vi "FK.vi"(8 "error in (no error)":errorcluster, 10 "joints":dbl[](array[numeric]), 11 "Delta Robot Kinematics in":refnum<class "Delta Robot Kinematics.lvclass">) -> (0 "error out":errorcluster, 1 "exist":bool, 2 "p":dbl[](array[numeric]), 3 "Delta Robot Kinematics out":refnum<class "Delta Robot Kinematics.lvclass">)   [LabVIEW 2014, in "Delta Robot Kinematics.lvclass"]
uses:
  Delta Robot Kinematics.lvclass
  Delta Robot Kinematics.lvclass/Delta Robot Kinematics.ctl
  <vilib>/Analysis/baseanly.llb/A x Vector.vi
  <vilib>/Analysis/_algsub.llb/Real Vector Norm.vi
  <vilib>/Analysis/baseanly.llb/Outer Product.vi
  <vilib>/Analysis/baseanly.llb/Real Outer Product.vi
  <vilib>/robotics/Kinematics/Create Lie Group Matrix.vi
  <vilib>/Analysis/7linalg.llb/Create Special Matrix.vi
  <vilib>/Analysis/7linalg.llb/Create Special Real Matrix.vi
  <vilib>/Analysis/Matrix/Numeric/Multiply/Multiply.vi
  <vilib>/Analysis/Matrix/Numeric/Multiply/Multiply - RM,R.vi
  <vilib>/Analysis/Matrix/Numeric/Multiply/Multiply - R,RM.vi
  <vilib>/Analysis/Matrix/Numeric/Add/Add.vi
  <vilib>/Analysis/Matrix/Numeric/Add/Add - RM,RM.vi
  <vilib>/robotics/Kinematics/NI_Kinematics.lvlib
  <vilib>/Analysis/NI_AALBase.lvlib
  <vilib>/Analysis/NI_AALPro.lvlib
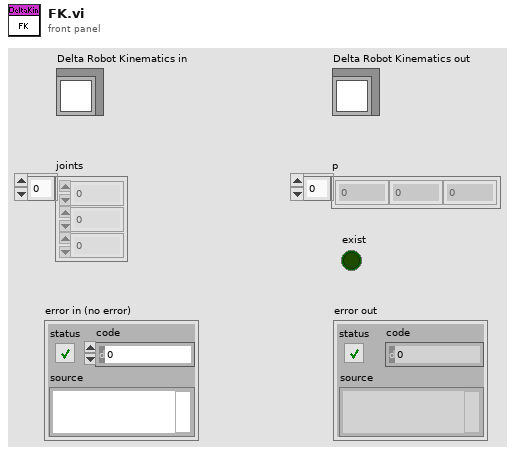
[diagram p1: front panel]
types:
  T1 = typedef "NI_Matrix.lvlib/RealMatrix.ctl" = dbl[][]
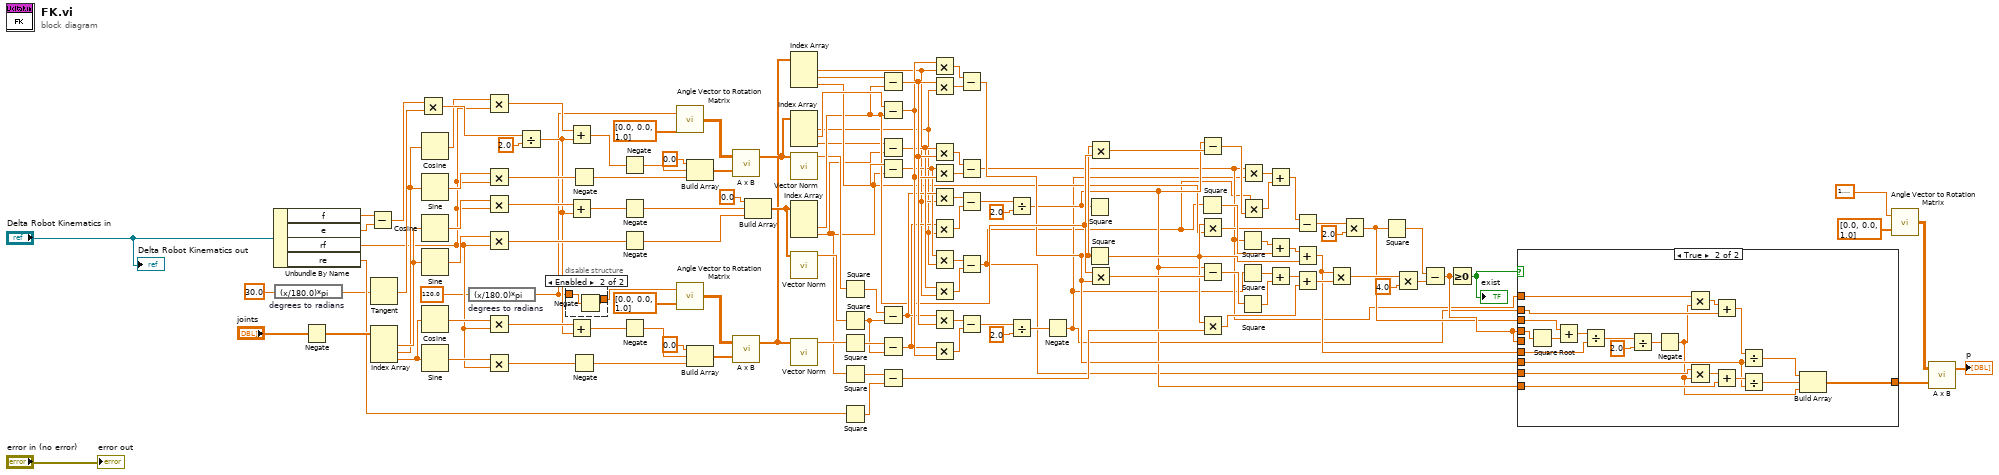
[diagram p0: block diagram]
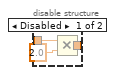
[diagram p2: hidden frame]
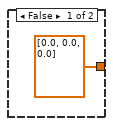
[diagram p3: hidden frame]
diagram:
  n1 = Unbundle By Name("Delta Robot Kinematics in") -> ("f"=w11:dbl, "e"=w10:dbl, "rf"=w9:dbl, "re"=w8:dbl)
  n2 = expression code="(x/180.0)*pi" "degrees to radians"(30.0) -> (w6:dbl)
  n3 = Negate(x="joints") -> (-x=w30:dbl[])
  n4 = Subtract(x=w11, y=w10) -> (x-y=w128:dbl)
  n5 = Tangent(1:w6) -> (0:w127:dbl)
  n6 = Index Array(array=w30) -> (element #1=w121:dbl, element #2=w51:dbl, element #3=w50:dbl)  [unwired: 3 in]
  n7 = Multiply(x=w128, y=w127) -> (x*y=w126:dbl)
  n8 = Cosine(x=w51) -> (cos(x)=w37:dbl)
  n9 = Sine(x=w51) -> (sin(x)=w35:dbl)
  n10 = Cosine(x=w121) -> (cos(x)=w124:dbl)
  n11 = Sine(x=w121) -> (sin(x)=w120:dbl)
  n12 = Cosine(x=w50) -> (cos(x)=w36:dbl)
  n13 = Sine(x=w50) -> (sin(x)=w33:dbl)
  n14 = expression code="(x/180.0)*pi" "degrees to radians"(120.0) -> (w4:dbl)
  n15 = Multiply(x=w37, y=w9) -> (x*y=w49:dbl)
  n16 = Multiply(x=w35, y=w9) -> (x*y=w47:dbl)
  n17 = Multiply(x=w124, y=w9) -> (x*y=w123:dbl)
  n18 = Multiply(x=w120, y=w9) -> (x*y=w119:dbl)
  n19 = Multiply(x=w36, y=w9) -> (x*y=w38:dbl)
  n20 = Multiply(x=w33, y=w9) -> (x*y=w40:dbl)
  n21 = Divide(x=w126, y=2.0) -> (x/y=w34:dbl)
  n22 = disable-structure shown="Enabled" {
    disable-tunnel: [w131 w133] -> w27
    disable-tunnel: w4 -> [w130 w134]
    frame Disabled {
      n23 = Multiply(x=w130, y=2.0) -> (x*y=w131:dbl)
    }
    frame Enabled {
      n24 = Negate(x=w134) -> (-x=w133:dbl)
    }
  }
  n25 = Add(x=w49, y=w34) -> (x+y=w48:dbl)
  n26 = Add(x=w123, y=w34) -> (x+y=w122:dbl)
  n27 = Add(x=w38, y=w34) -> (x+y=w39:dbl)
  n28 = Negate(x=w47) -> (-x=w45:dbl)
  n29 = Negate(x=w40) -> (-x=w42:dbl)
  n30 = Negate(x=w48) -> (-x=w46:dbl)
  n31 = Negate(x=w122) -> (-x=w118:dbl)
  n32 = Negate(x=w119) -> (-x=w117:dbl)
  n33 = Negate(x=w39) -> (-x=w41:dbl)
  n34 = call <vilib>:"Angle Vector to Rotation Matrix.vi"("vector"=dbl[] [0.0, 0.0, 1.0], "angle"=w4) -> ("rotation matrix"=w114:T1)
  n35 = call <vilib>:"Angle Vector to Rotation Matrix.vi"("vector"=dbl[] [0.0, 0.0, 1.0], "angle"=w27) -> ("rotation matrix"=w28:T1)
  n36 = Build Array(0.0 ("element"), w46, w45) -> (w32:dbl[])
  n37 = Build Array(0.0 ("element"), w41, w42) -> (w31:dbl[])
  n38 = call-poly <vilib>:"A x B.vi"("Vector"=w32, "A"=w114) -> ("A x Vector"=w108:dbl[])  [unwired: 1 out]
  n39 = call-poly <vilib>:"A x B.vi"("Vector"=w31, "A"=w28) -> ("A x Vector"=w107:dbl[])  [unwired: 1 out]
  n40 = Build Array(0.0 ("element"), w118, w117) -> (w109:dbl[])
  n41 = Index Array(array=w107) -> (element #1=w90:dbl, element #2=w111:dbl, element #3=w105:dbl)  [unwired: 3 in]
  n42 = Index Array(array=w108) -> (element #1=w19:dbl, element #2=w113:dbl, element #3=w20:dbl)  [unwired: 3 in]
  n43 = call-poly <vilib>:"Vector Norm.vi"("Input Vector"=w108) -> ("norm"=w24:dbl)  [unwired: 9 in, 1 out]
  n44 = Index Array(array=w109) -> (element #2=w75:dbl, element #3=w18:dbl)  [unwired: 3 in, 1 out]
  n45 = call-poly <vilib>:"Vector Norm.vi"("Input Vector"=w109) -> ("norm"=w22:dbl)  [unwired: 9 in, 1 out]
  n46 = call-poly <vilib>:"Vector Norm.vi"("Input Vector"=w107) -> ("norm"=w26:dbl)  [unwired: 9 in, 1 out]
  n47 = Square(x=w24) -> (x^2=w23:dbl)
  n48 = Square(x=w22) -> (x^2=w21:dbl)
  n49 = Square(x=w26) -> (x^2=w25:dbl)
  n50 = Square(x=w18) -> (x^2=w70:dbl)
  n51 = Square(x=w8) -> (x^2=w69:dbl)
  n52 = Subtract(x=w111, y=w75) -> (x-y=w103:dbl)
  n53 = Subtract(x=w113, y=w75) -> (x-y=w102:dbl)
  n54 = Subtract(x=w20, y=w18) -> (x-y=w96:dbl)
  n55 = Subtract(x=w105, y=w18) -> (x-y=w92:dbl)
  n56 = Subtract(x=w23, y=w21) -> (x-y=w93:dbl)
  n57 = Subtract(x=w25, y=w21) -> (x-y=w91:dbl)
  n58 = Subtract(x=w70, y=w69) -> (x-y=w68:dbl)
  n59 = Multiply(x=w102, y=w90) -> (x*y=w112:dbl)
  n60 = Multiply(x=w103, y=w19) -> (x*y=w110:dbl)
  n61 = Multiply(x=w96, y=w103) -> (x*y=w106:dbl)
  n62 = Multiply(x=w92, y=w102) -> (x*y=w104:dbl)
  n63 = Multiply(x=w93, y=w90) -> (x*y=w89:dbl)
  n64 = Multiply(x=w91, y=w19) -> (x*y=w88:dbl)
  n65 = Multiply(x=w92, y=w19) -> (x*y=w95:dbl)
  n66 = Multiply(x=w96, y=w90) -> (x*y=w94:dbl)
  n67 = Multiply(x=w93, y=w103) -> (x*y=w101:dbl)
  n68 = Multiply(x=w91, y=w102) -> (x*y=w100:dbl)
  n69 = Subtract(x=w112, y=w110) -> (x-y=w59:dbl)
  n70 = Subtract(x=w106, y=w104) -> (x-y=w17:dbl)
  n71 = Subtract(x=w89, y=w88) -> (x-y=w87:dbl)
  n72 = Subtract(x=w95, y=w94) -> (x-y=w2:dbl)
  n73 = Subtract(x=w101, y=w100) -> (x-y=w99:dbl)
  n74 = Divide(x=w87, y=2.0) -> (x/y=w58:dbl)
  n75 = Divide(x=w99, y=2.0) -> (x/y=w97:dbl)
  n76 = Negate(x=w97) -> (-x=w16:dbl)
  n77 = Square(x=w58) -> ()  [unwired: 1 out]
  n78 = Square(x=w59) -> (x^2=w67:dbl)
  n79 = Multiply(x=w59, y=w75) -> (x*y=w83:dbl)
  n80 = Multiply(x=w75, y=w59) -> (x*y=w74:dbl)
  n81 = Square(x=w2) -> (x^2=w81:dbl)
  n82 = Subtract(x=w58, y=w83) -> (x-y=w82:dbl)
  n83 = Multiply(x=w67, y=w18) -> (x*y=w78:dbl)
  n84 = Subtract(x=w58, y=w74) -> (x-y=w73:dbl)
  n85 = Multiply(x=w67, y=w68) -> (x*y=w65:dbl)
  n86 = Square(x=w17) -> (x^2=w85:dbl)
  n87 = Square(x=w16) -> (x^2=w72:dbl)
  n88 = Square(x=w73) -> (x^2=w71:dbl)
  n89 = Multiply(x=w17, y=w16) -> (x*y=w15:dbl)
  n90 = Multiply(x=w2, y=w82) -> (x*y=w80:dbl)
  n91 = Add(x=w15, y=w80) -> (x+y=w79:dbl)
  n92 = Add(x=w85, y=w81) -> (x+y=w84:dbl)
  n93 = Add(x=w72, y=w71) -> (x+y=w66:dbl)
  n94 = Subtract(x=w79, y=w78) -> (x-y=w77:dbl)
  n95 = Add(x=w84, y=w67) -> (x+y=w55:dbl)
  n96 = Add(x=w66, y=w65) -> (x+y=w64:dbl)
  n97 = Multiply(x=w55, y=w64) -> (x*y=w63:dbl)
  n98 = Multiply(x=w77, y=2.0) -> (x*y=w56:dbl)
  n99 = Square(x=w56) -> (x^2=w61:dbl)
  n100 = Multiply(x=w63, y=4.0) -> (x*y=w60:dbl)
  n101 = Subtract(x=w61, y=w60) -> (x-y=w57:dbl)
  n102 = Greater Or Equal To 0?(x=w57) -> (x >= 0?=w13:bool)
  "exist" <- w13
  n103 = case shown="True" w13 {
    tunnel: w57 -> [_ _]
    tunnel: w17 -> [_ w156]
    tunnel: w16 -> [_ w154]
    tunnel: w59 -> [_ w148]
    tunnel: w2 -> [_ w152]
    tunnel: w58 -> [_ w150]
    tunnel: w57 -> [_ w147]
    tunnel: w56 -> [_ w145]
    tunnel: w55 -> [_ w143]
    tunnel: [dbl[] [0.0, 0.0, 0.0] w140] -> w52
    frame False {
    }
    frame True {
      n104 = Square Root(x=w147) -> (sqrt(x)=w146:dbl)
      n105 = Add(x=w145, y=w146) -> (x+y=w144:dbl)
      n106 = Divide(x=w144, y=w143) -> (x/y=w142:dbl)
      n107 = Divide(x=w142, y=2.0) -> (x/y=w139:dbl)
      n108 = Negate(x=w139) -> (-x=w138:dbl)
      n109 = Multiply(x=w156, y=w138) -> (x*y=w155:dbl)
      n110 = Multiply(x=w152, y=w138) -> (x*y=w151:dbl)
      n111 = Add(x=w155, y=w154) -> (x+y=w153:dbl)
      n112 = Add(x=w151, y=w150) -> (x+y=w149:dbl)
      n113 = Divide(x=w153, y=w148) -> (x/y=w137:dbl)
      n114 = Divide(x=w149, y=w148) -> (x/y=w136:dbl)
      n115 = Build Array(w137, w136, w138) -> (w140:dbl[])
    }
  }
  n116 = call <vilib>:"Angle Vector to Rotation Matrix.vi"("vector"=dbl[] [0.0, 0.0, 1.0], "angle"=1.5707963267948966) -> ("rotation matrix"=w53:T1)
  n117 = call-poly <vilib>:"A x B.vi"("Vector"=w52, "A"=w53) -> ("A x Vector"=→"p":dbl[])  [unwired: 1 out]
  "Delta Robot Kinematics out" <- "Delta Robot Kinematics in"
  "error out" <- "error in (no error)"
